vi "SbigMisc.vi"(4 "Misc":cluster{"Fan":u16, "Shutter":u16, "Led":u16} {"Led" items=["OFF", "ON", "BLINK LOW", "BLINK HIGH"]; "Shutter" items=["LEAVE", "OPEN", "CLOSE", "REINIT"]; "Fan" items=["OFF", "ON"]}, 5 "SbigReference":T1, 6 "error in (no error)":errorcluster) -> (0 "error out":errorcluster)   [LabVIEW 2009]
uses:
  Controls/SbigReference.ctl
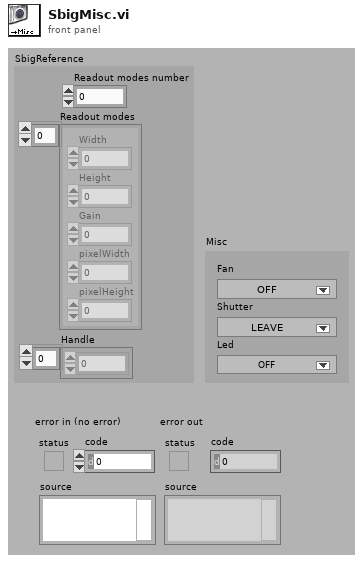
[diagram p1: front panel]
types:
  T1 = typedef "SbigReference.ctl" = cluster{"Readout modes number":u16, "Readout modes":cluster{"Width":u16, "Height":u16, "Gain":dbl, "pixelWidth":dbl, "pixelHeight":dbl}[], "Handle":u16[]}
  T2 = enum16{"0-NoCommand", "1-StartExposure", "2-EndExposure", "3-ReadoutLine", "4-DumpLines", "5-SetTemperatureRegulation", "6-QueryTemperatureStatus", "7-ActivateRelay", "8-PulseOut", "9-EstablishLink", "10-GetDriverInfo", "11-GetCCDInfo", "12-QueryCommandStatus", "13-MiscellaneousControl", "14-ReadSubstractLine", "15-UpdateClock", "16-ReadOffset", "17-OpenDriver", "18-CloseDriver", "19-TXSerialBytes", "20-GetSerialStatus", "21-AOTipTilt", "22-AOSetFocus", "23-AODelay", "24-GetTurboStatus", "25-EndReadout", "26-GetUSTimer", "27-OpenDevice", "28-CloseDevice", "29-SetIRQL", "30-GetIRQL", "31-GetLine", "32-GetLinkStatus", "33-GetDriverHandle", "34-SetDriverHandle", "35-StartReadout", "36-GetErrorString", "37-SetDriverControl", "38-GetDriverControl", "39-USBADControl", "40-QueryUSB", "41-GetPentiumCycleCount", "42-RWUSBI2C", "43-CFW"}
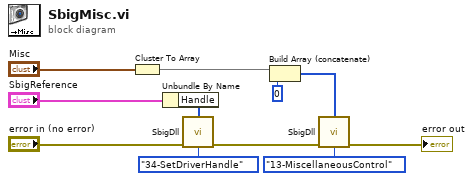
[diagram p0: block diagram]
diagram:
  n1 = Cluster To Array(cluster="Misc") -> (array=w2:u16[])
  n2 = Unbundle By Name("SbigReference") -> ("Handle"=w4:u16[])
  n3 = call "SbigDll.vi"("error in (no error)"="error in (no error)", "Command"=T2."34-SetDriverHandle", "Parameters"=w4) -> ("error out"=w5:errorcluster)  [unwired: 1 in, 3 out]
  n4 = Build Array (concatenate)(w2, u16 0) -> (w9:u16[])
  n5 = call "SbigDll.vi"("error in (no error)"=w5, "Command"=T2."13-MiscellaneousControl", "Parameters"=w9) -> ("error out"=→"error out":errorcluster)  [unwired: 1 in, 3 out]
